vi "PR_All.vi"(8 "error in (no error)":errorcluster, 11 "DBlink":string="Driver={ODBC Driver 17 for SQL Server};Server=localhost\\SQLEXPRESS;Database=ZDX201;UID=labview;PWD=Dsa@54137926") -> (0 "error out":errorcluster={"status"=TRUE, "code"=-2147217843, "source"="NI_Database_API.lvlib:DB Tools Open Connec (String).vi->WD_assemble_data.vi<ERR>ADO Error: 0x80040E4D\r\nException occured in Microsoft OLE DB Provider for ODBC Drivers: [Microsoft][ODBC Driver 17 for SQL Server][SQL Server]使用者 'labview' 的登入失敗。 in NI_Database_API.lvlib:DB Tools Open Connec (String).vi->WD_assemble_data.vi"}, 3 "Production":T1(array[cluster]))   [LabVIEW 2019]
uses:
  <vilib>/addons/database/Connection.llb/DB Tools Open Connec (String).vi
  <vilib>/addons/database/Connection.llb/Conn Execute.vi
  <vilib>/addons/database/Recordset.llb/Rec Fetch Recordset Data (R).vi
  <vilib>/addons/database/Recordset.llb/Rec Destroy - Connection.vi
  <vilib>/addons/database/_DB Variant To Data/Database Variant To Data.xnode
  <vilib>/addons/database/NI_Database_API.lvlib
panel:
  out "查詢結果":string="SELECT [id]\n      ,[name]\n      ,[barcode A]\n      ,[barcode B]\n      ,[update_time]\n  FROM [ZDX201].[dbo].[workplace_data]\n  where id>0 and id<6\n  order by id"
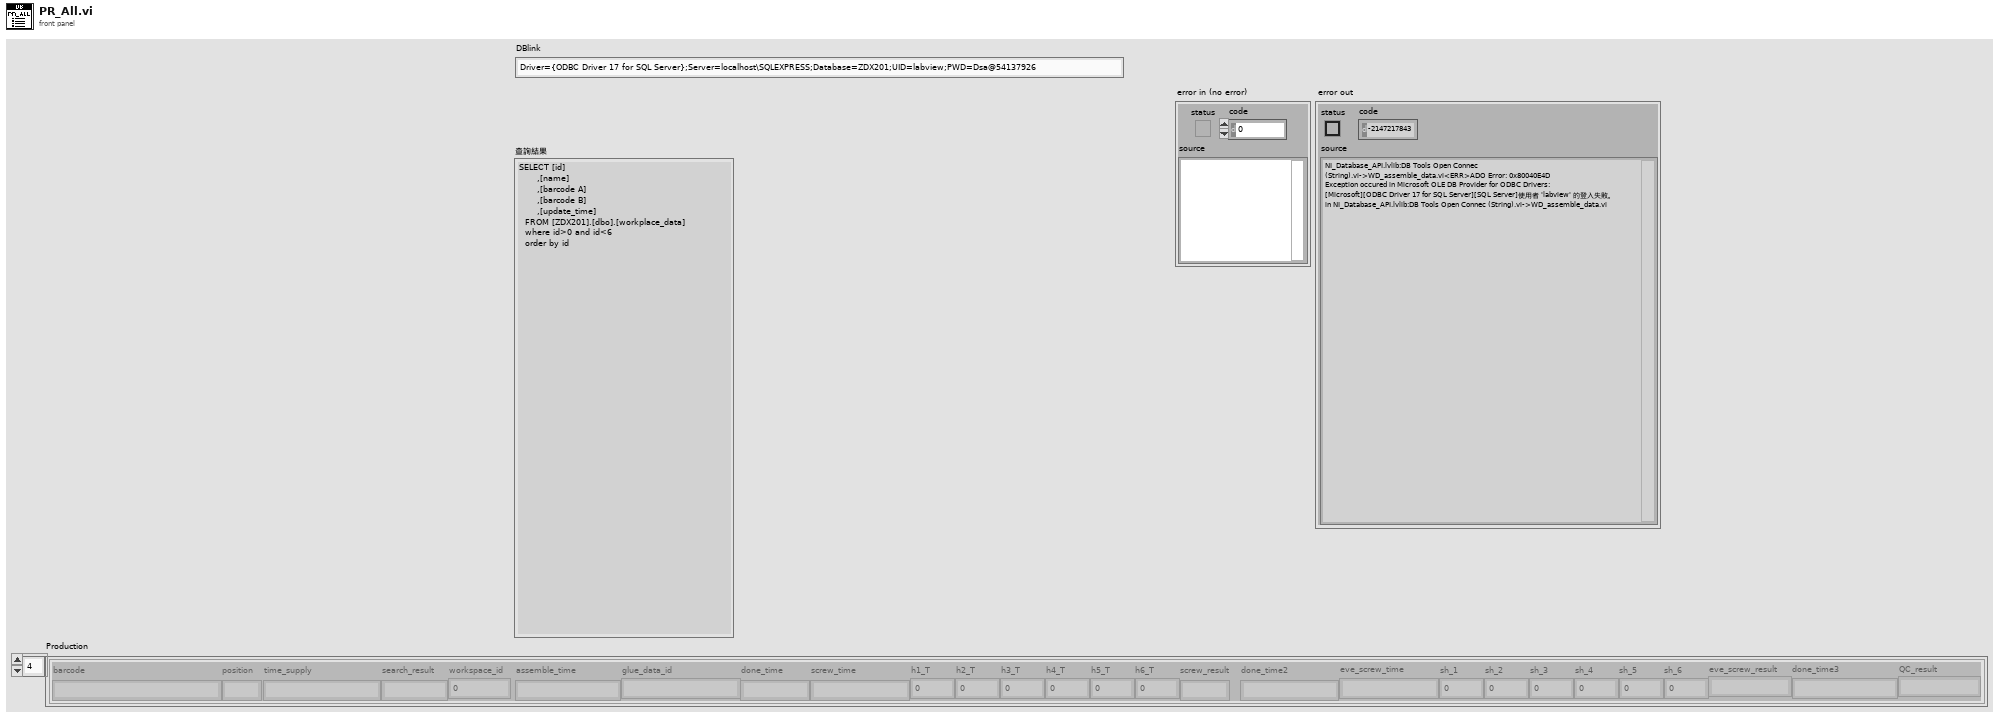
[diagram p1: front panel]
types:
  T1 = cluster{"barcode":string, "position":string, "time_supply":string, "search_result":string, "workspace_id":i16, "assemble_time":string, "glue_data_id":string, "done_time":string, "screw_time":string, "h1_T":dbl, "h2_T":dbl, "h3_T":dbl, "h4_T":dbl, "h5_T":dbl, "h6_T":dbl, "screw_result":string, "done_time2":string, "eve_screw_time":string, "sh_1":dbl, "sh_2":dbl, "sh_3":dbl, "sh_4":dbl, "sh_5":dbl, "sh_6":dbl, "eve_screw_result":string, "done_time3":string, "QC_result":string}[]
  T2 = typedef "NI_Database_API.lvlib/Conn ObjectReference.ctl" = refnum<k1>
  T3 = typedef "NI_Database_API.lvlib/Rec ObjectReference.ctl" = refnum<k1>
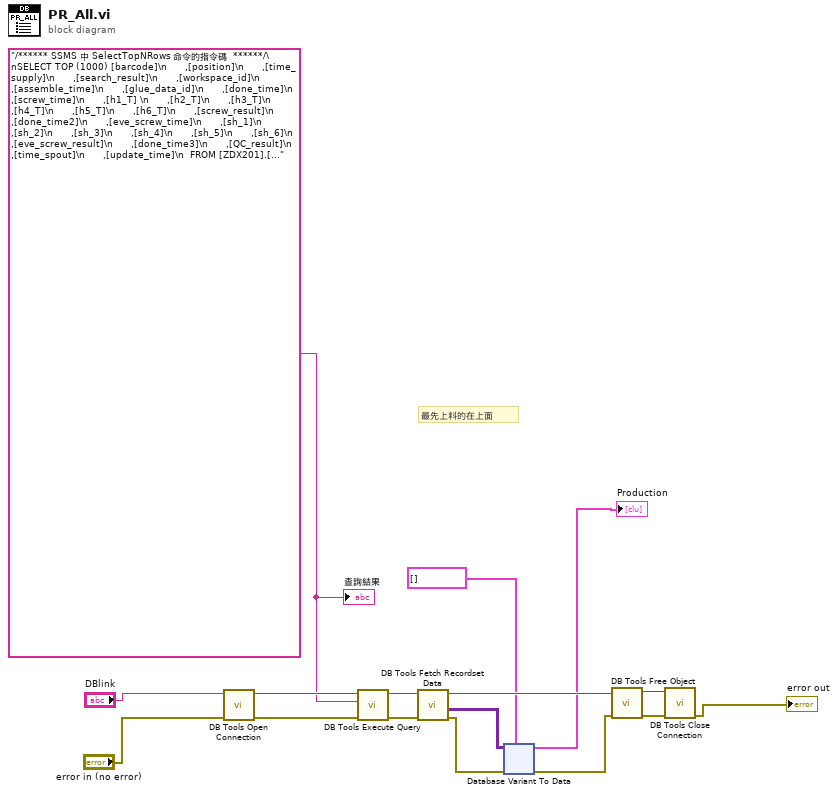
[diagram p0: block diagram]
diagram:
  w7 = "/****** SSMS 中 SelectTopNRows 命令的指令碼  ******/\nSELECT TOP (1000) [barcode]\n      ,[position]\n      ,[time_supply]\n      ,[search_result]\n      ,[workspace_id]\n      ,[assemble_time]\n      ,[glue_data_id]\n      ,[done_time]\n      ,[screw_time]\n      ,[h1_T] \n      ,[h2_T]\n      ,[h3_T]\n      ,[h4_T]\n      ,[h5_T]\n      ,[h6_T]\n      ,[screw_result]\n      ,[done_time2]\n      ,[eve_screw_time]\n      ,[sh_1]\n      ,[sh_2]\n      ,[sh_3]\n      ,[sh_4]\n      ,[sh_5]\n      ,[sh_6]\n      ,[eve_screw_result]\n      ,[done_time3]\n      ,[QC_result]\n      ,[time_spout]\n      ,[update_time]\n  FROM [ZDX201].[dbo].[production]\n  order by time_supply asc"
  # "最先上料的在上面"
  n1 = call-poly <vilib>:"DB Tools Open Connection.vi"("error in (no error)"="error in (no error)", "connection information"="DBlink") -> ("error out"=w16:errorcluster, "connection reference"=w15:T2)  [unwired: 6 in]
  n2 = call-poly <vilib>:"DB Tools Execute Query.vi"("error in (no error)"=w16, "SQL query"=w7, "connection reference"=w15) -> ("error out"=w13:errorcluster, "recordset reference"=w14:T3)  [unwired: 5 in]
  n3 = call-poly <vilib>:"DB Tools Fetch Recordset Data.vi"("error in (no error)"=w13, "recordset reference"=w14) -> ("error out"=w8:errorcluster, "recordset data"=w1:variant[][], "recordset reference out"=w9:T3)  [unwired: 3 in]
  n4 = xnode "Database Variant To Data"("database variant"=w1, "error in (no error)"=w8, "type"=T1 [] ("Production")) -> ("data"=→"Production":T1, "error out"=w10:errorcluster)
  n5 = call-poly <vilib>:"DB Tools Free Object.vi"("error in (no error)"=w10, "recordset reference"=w9) -> ("error out"=w11:errorcluster, "connection reference"=w12:T2)  [unwired: 8 in]
  n6 = call <vilib>:"DB Tools Close Connection.vi"("error in (no error)"=w11, "connection reference"=w12) -> ("error out"=→"error out":errorcluster)  [unwired: 5 in]
  "查詢結果" <- w7
